vi "AddDependenciesOfLibrary.vi"(8 "error in (no error)":errorcluster, 9 "LibraryName":string="ModuleA", 10 "Project Path":path=path "E:/sw-deps-monitor/Source/BuildSpecs/Modules/ModuleA.lvproj", 11 "Config Refnum in":T1) -> (0 "error out":errorcluster, 2 "ActualDependencies":string[](array[string]), 3 "Config Refnum out":T1)   [LabVIEW 2023, in "DepsWatch.lvlib"]
uses:
  DepsWatch.lvlib
  <vilib>/Utility/config.llb/Config Data RefNum.ctl
  <vilib>/Utility/config.llb/Write Key (String).vi
  <vilib>/Utility/config.llb/NI_LVConfig.lvlib
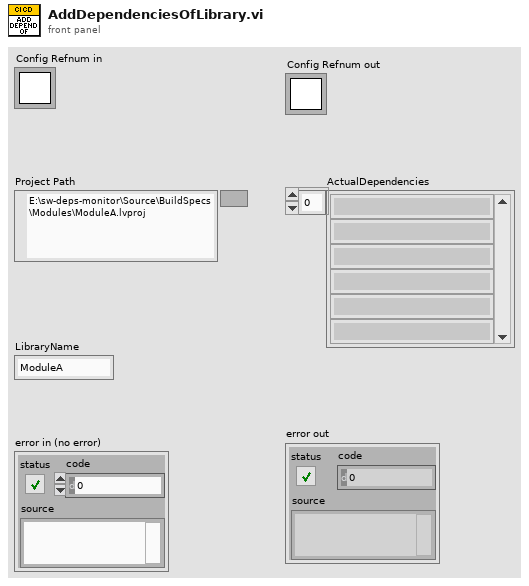
[diagram p1: front panel]
types:
  T1 = typedef "NI_LVConfig.lvlib/Config Data RefNum.ctl" = refnum<k1>
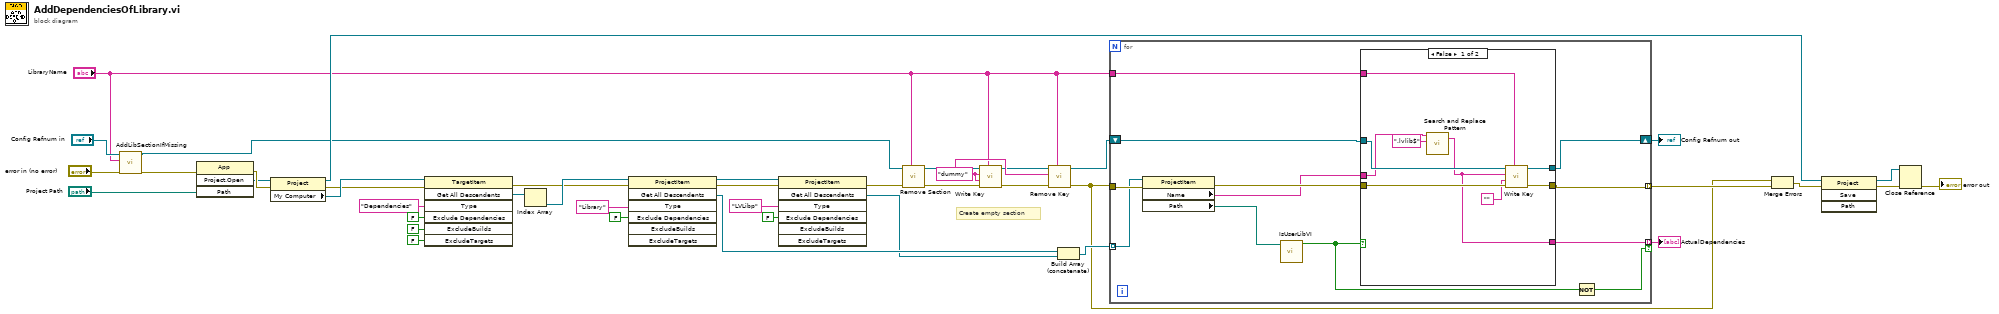
[diagram p0: block diagram]
diagram:
  w6 = "dummy" ("key")
  # "Create empty section"
  n1 = call "AddLibSectionIfMissing.vi"("error in (no error)"="error in (no error)", "LibraryName"="LibraryName", "Config Refnum in"="Config Refnum in") -> ("error out"=w13:errorcluster, "Config Refnum out"=w9:T1)  [unwired: 7 in]
  n2 = invoke class="App" method="Project.Open"(error in=w13, "Path"="Project Path") -> (error out=w41:errorcluster, "Project:Open"=w40:refnum<vi>)  [unwired: 2 in, 2 out]
  n3 = property class="Project"(reference=w40, error in=w41) -> (reference out=w25:refnum<vi>, error out=w28:errorcluster, "My Computer"=w34:refnum<vi>)
  n4 = invoke class="TargetItem" method="Get All Descendents"(reference=w34, error in=w28, "Type"="Dependencies", "Exclude Dependencies"=FALSE ("ExcludeDependencies"), "ExcludeBuilds"=FALSE, "ExcludeTargets"=FALSE) -> (error out=w27:errorcluster, "All Descendents"=w30:refnum<vi>[])  [unwired: 1 in, 5 out]
  n5 = Index Array(array=w30) -> (element=w29:refnum<vi>)  [unwired: 1 in]
  n6 = invoke class="ProjectItem" method="Get All Descendents"(reference=w29, error in=w27, "Type"="Library", "Exclude Dependencies"=FALSE ("ExcludeDependencies")) -> (reference out=w20:refnum<vi>, error out=w21:errorcluster, "All Descendents"=w17:refnum<vi>[])  [unwired: 3 in, 4 out]
  n7 = invoke class="ProjectItem" method="Get All Descendents"(reference=w20, error in=w21, "Type"="LVLibp", "Exclude Dependencies"=FALSE ("ExcludeDependencies")) -> (error out=w10:errorcluster, "All Descendents"=w16:refnum<vi>[])  [unwired: 3 in, 5 out]
  n8 = call <vilib>:"Remove Section.vi"("section"="LibraryName", "error in (no error)"=w10, "refnum"=w9) -> ("error out"=w8:errorcluster, "refnum out"=w7:T1)  [unwired: 6 in, 1 out]
  n9 = call-poly <vilib>:"Write Key.vi"("section"="LibraryName", "error in (no error)"=w8, "value"=w6, "key"=w6, "refnum"=w7) -> ("error out"=w5:errorcluster, "refnum out"=w4:T1)  [unwired: 4 in, 1 out]
  n10 = call <vilib>:"Remove Key.vi"("section"="LibraryName", "error in (no error)"=w5, "key"=w6, "refnum"=w4) -> ("error out"=w1:errorcluster, "refnum out"=w3:T1)  [unwired: 5 in, 1 out]
  n11 = Build Array (concatenate)(w17, w16) -> (w15:refnum<vi>[])
  n12 = for {
    tunnel: w1 -> [w54]
    tunnel: w15 -> [w47] mode=indexing
    tunnel: "LibraryName" -> [w51]
    tunnel: [w48] -> w39 mode=indexing
    shift-right: [w49] -> w38
    shift-left: w3 -> [w53]
    tunnel: [w45] -> w11 mode=indexing if=w43
    n13 = property class="ProjectItem"(reference=w47, error in=w54) -> (error out=w52:errorcluster, "Name"=w50:string, "Path"=w46:path)  [unwired: 1 out]
    n14 = call "IsUserLibVI.vi"("ItemPath"=w46) -> ("IsUserLibVI?"=w44:bool)  [unwired: 10 in]
    n15 = case shown="False" w44 {
      tunnel: w53 -> [w62 w64]
      tunnel: w52 -> [w63 w65]
      tunnel: w51 -> [w61 _]
      tunnel: w50 -> [w58 _]
      tunnel: [w57 w65] -> w48
      tunnel: [w56 w64] -> w49
      tunnel: [w55 _] -> w45
      frame False {
        n16 = call <vilib>:"Search and Replace Pattern.vi"("string"=w58, "regular expression (\"\")"=".lvlib$" ("regular expression (\"\")")) -> ("result string"=w55:string)  [unwired: 3 in, 1 out]
        n17 = call-poly <vilib>:"Write Key.vi"("section"=w61, "error in (no error)"=w63, "value"="", "key"=w55, "refnum"=w62) -> ("error out"=w57:errorcluster, "refnum out"=w56:T1)  [unwired: 4 in, 1 out]
      }
      frame True {
      }
    }
    n18 = Not(x=w44) -> (.not. x?=w43:bool)
  }
  "Config Refnum out" <- w38
  "ActualDependencies" <- w11
  n19 = Merge Errors(w1, w39) -> (w26:errorcluster)
  n20 = invoke class="Project" method="Save"(reference=w25, error in=w26) -> (reference out=w24:refnum<vi>, error out=w23:errorcluster)  [unwired: 2 in, 2 out]
  n21 = Close Reference(reference=w24, error in (no error)=w23) -> (error out=→"error out":errorcluster)
